vi "Parsing_TheGooodOne.vi"(6 "array":dbl[](array[numeric])=[0.0], 7 "Iterations":i32=6079, 8 "Search_Params":string[](array[string])=["B", "X", "Y", "W1", "H1", "W2", "H2"], 9 "Input":string="B:0,X:-3,Y:-3,W1:-3,H1:-3,W2:-3,H2:-3") -> (2 "Corrected distance":dbl=-10000.0, 3 "Value-Reference":dbl=-292.57472985881094)   [LabVIEW 2016]
uses:
  <vilib>/Analysis/3filter.llb/IIR Filter (DBL).vi
  <vilib>/Analysis/NI_AALBase.lvlib
panel:
  in  "Bad Value Count":i32=4
  out "Waveform Chart":cluster{dbl, dbl}(graph)={-10000.0, -292.57472985881094}
  out "Positions 2":i32[](array[numeric])
  out "Distance":dbl=133.35829999999999
  out "Move left":bool
  out "Move right":bool
  out "Not target":bool=TRUE
  in  "Desired_Midpoint":i32=200
  in  "High_Band":i32=10
  in  "Low_Band":i32=10
  out "Error":i32
  in  "P-gain":dbl format="%#_13g"
  out "Effort_Error":dbl
  out "Good_Midp":bool
  out "X Value":i32
  out "Good Target 2":bool
  out "Positions":i32[](array[numeric])
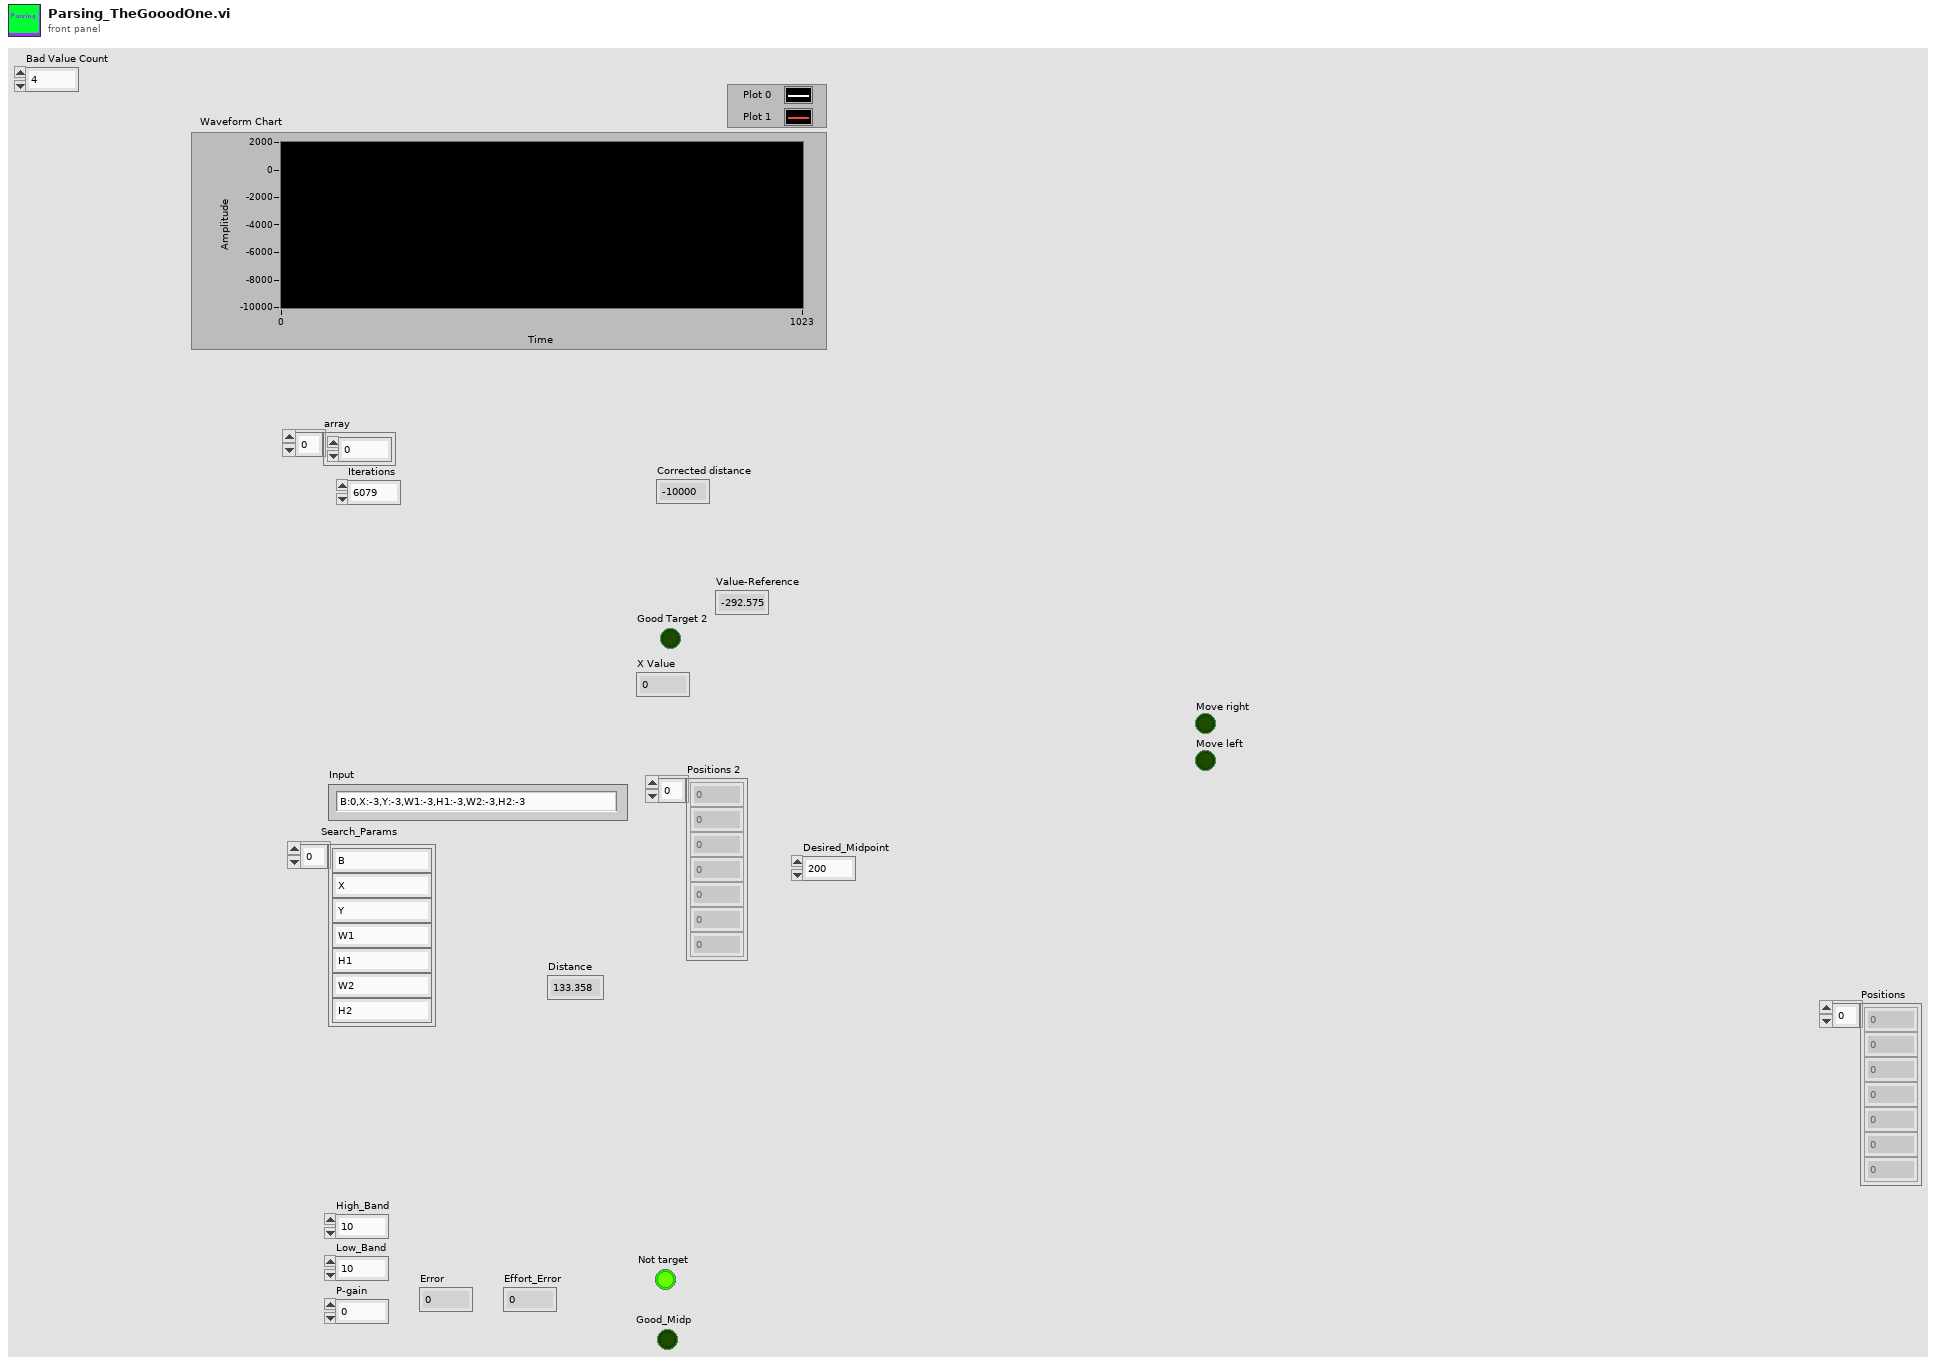
[diagram p1: front panel]
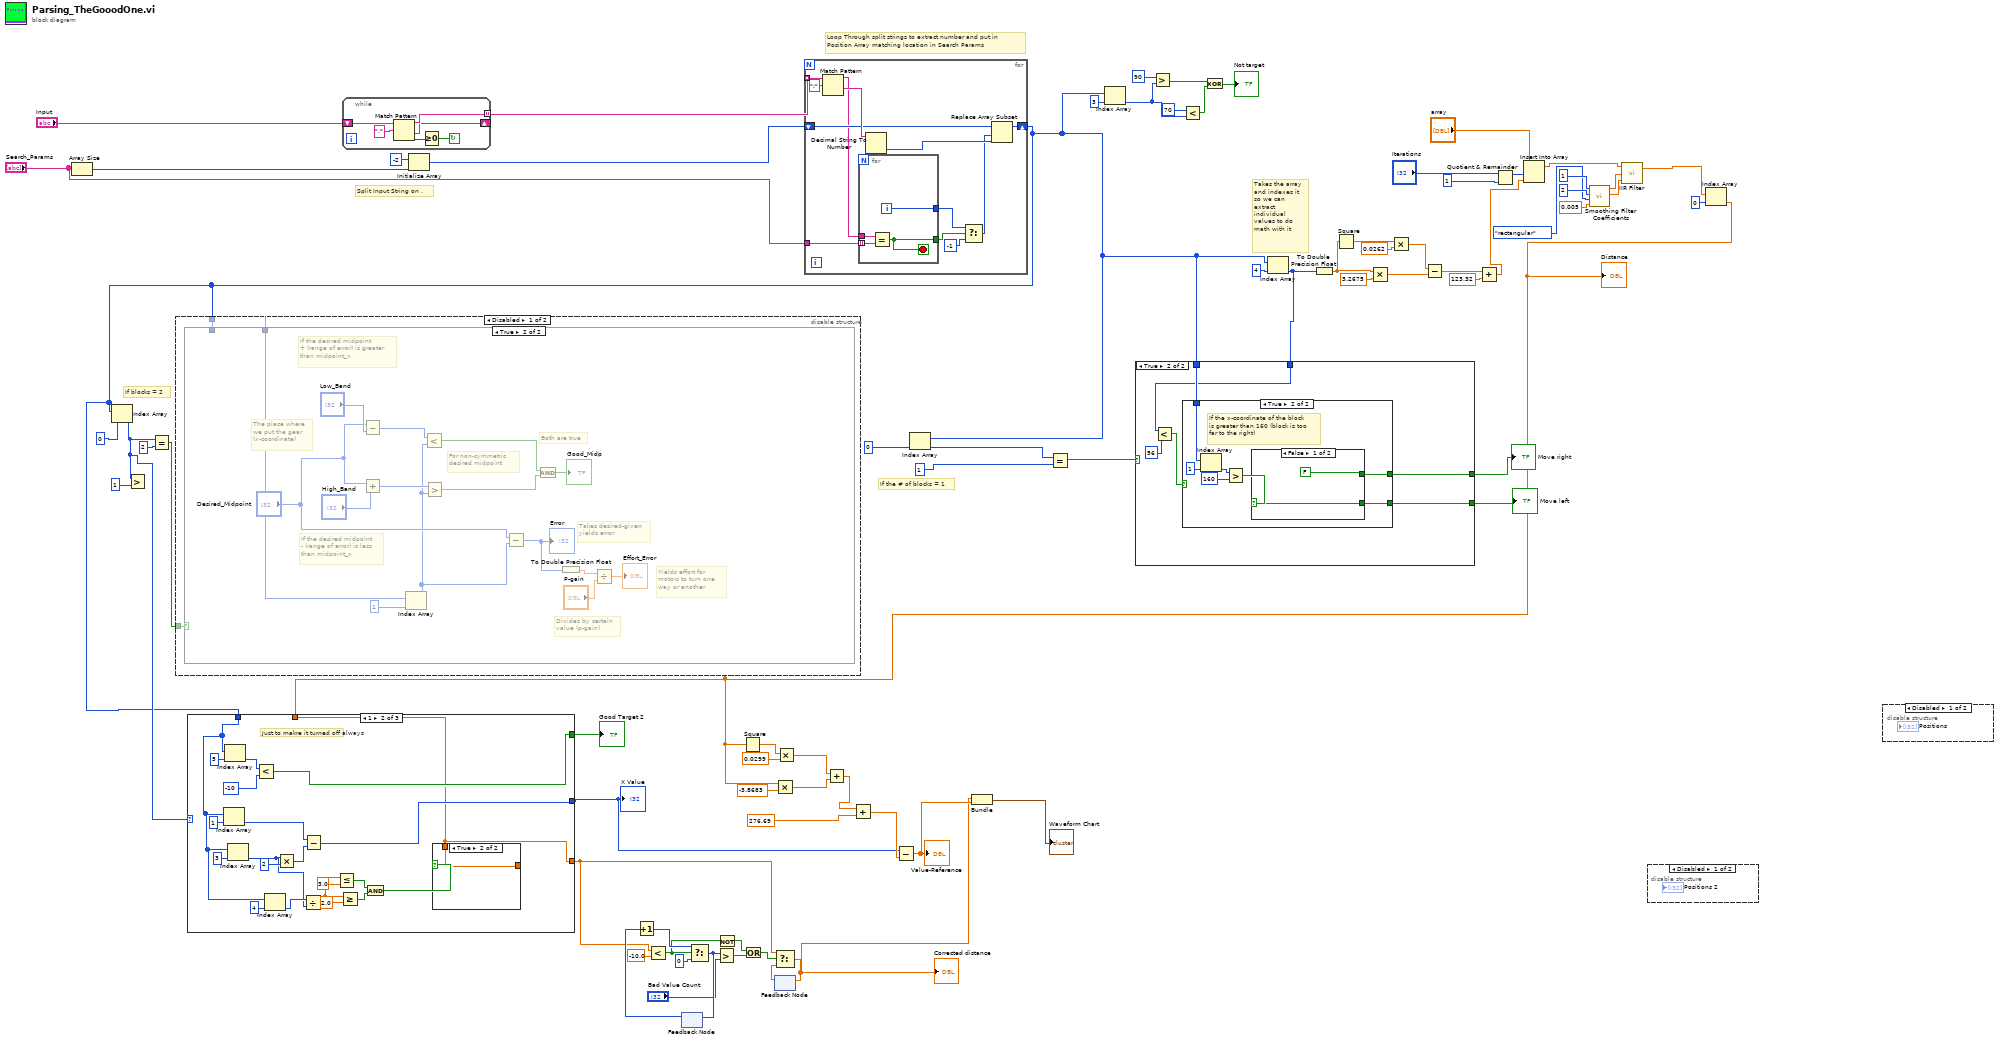
[diagram p0: block diagram]
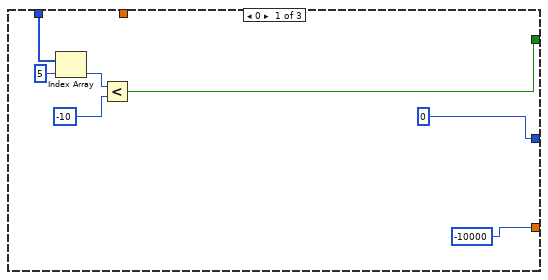
[diagram p2: hidden frame]
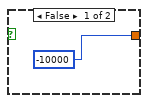
[diagram p3: hidden frame]
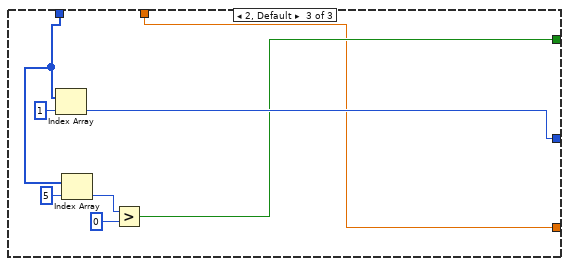
[diagram p4: hidden frame]
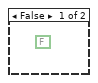
[diagram p5: hidden frame]
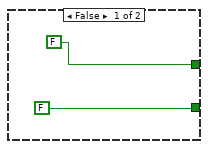
[diagram p7: hidden frame]
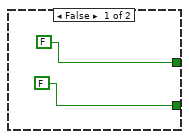
[diagram p8: hidden frame]
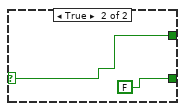
[diagram p9: hidden frame]
diagram:
  # "If blocks = 2"
  # "If the # of blocks = 1"
  # "Takes the array and indexes it so we can extract individual values to do math with it"
  # "Loop Through split strings to extract number and put in\nPosition Array matching location in Search Params"
  # "Split Input String on ,"
  n1 = Array Size(array="Search_Params") -> (size(s)=w36:i32)
  n2 = while {
    shift-right: [w78] -> _
    shift-left: "Input" -> [w81]
    tunnel: [w79] -> w32 mode=indexing
    stop <- w76 continue-if-true
    n3 = Match Pattern(string=w81, regular expression=",") -> (before substring=w79:string, after substring=w78:string, offset past match=w77:i32)  [unwired: 1 in, 1 out]
    n4 = Greater Or Equal To 0?(x=w77) -> (x >= 0?=w76:bool)
  }
  n5 = Initialize Array(-2 ("element"), w36) -> (w34:i32[])
  n6 = feedback #1() -> (w11:i32)  [unwired: 1 in]
  n7 = Increment(x=w11) -> (x+1=w12:i32)
  n8 = feedback #2() -> (w4:dbl)  [unwired: 1 in]
  n9 = for {
    tunnel: w32 -> [w93] mode=indexing
    shift-right: [w89] -> w64
    shift-left: w34 -> [w90]
    tunnel: "Search_Params" -> [w86]
    n10 = Match Pattern(string=w93, regular expression=":") -> (before substring=w87:string, after substring=w91:string)  [unwired: 1 in, 2 out]
    n11 = for {
      tunnel: w87 -> [w97]
      tunnel: w86 -> [w96] mode=indexing
      tunnel: [w94] -> w85
      tunnel: [w95] -> w84
      i -> [w95]
      stop <- w94 stop-if-true
      n12 = Equal?(x=w97, y=w96) -> (x = y?=w94:bool)
    }
    n13 = Decimal String To Number(string=w91) -> (number=w88:i32)  [unwired: 2 in, 1 out]
    n14 = Select(t=w84, s=w85, f=-1) -> (s? t:f=w82:i32)
    n15 = Replace Array Subset(array=w90, new element=w88, index=w82) -> (w89:i32[])
  }
  n16 = Index Array(array=w64, index=0) -> (element=w65:i32)
  n17 = Greater?(x=w65, y=1) -> ()  [unwired: 1 out]
  n18 = Equal?(x=w65, y=2) -> (x = y?=w55:bool)
  n19 = disable-structure shown="Disabled" {
    disable-tunnel: w55 -> [w99 _]
    disable-tunnel: w64 -> [w98 _]
    frame Disabled {
      n20 = case shown="True" w99 {
        tunnel: w98 -> [_ _]
        tunnel: w98 -> [_ w100]
        frame False {
          (unwired) FALSE
        }
        frame True {
          # "Yields effort for\nmotors to turn one\nway or another"
          # "Divides by certain\nvalue (p-gain)"
          # "Takes desired-given\nyields error"
          # "The place where\nwe put the gear \n(x-coordinate)"
          # "Both are true"
          # "For non-symmetric\ndesired midpoint"
          # "If the desired midpoint\n- (range of error) is less\nthan midpoint_x"
          # "If the desired midpoint\n+ (range of error) is greater\nthan midpoint_x"
          n21 = Subtract(x="Desired_Midpoint", y="Low_Band") -> (x-y=w110:i32)
          n22 = Add(x="Desired_Midpoint", y="High_Band") -> (x+y=w111:i32)
          n23 = Index Array(array=w100, index=1) -> (element=w106:i32)
          n24 = Less?(x=w110, y=w106) -> (x < y?=w109:bool)
          n25 = Greater?(x=w111, y=w106) -> (0:w108:bool)
          n26 = Subtract(x="Desired_Midpoint", y=w106) -> (x-y=w105:i32)
          "Error" <- w105
          n27 = And(x=w109, y=w108) -> (x .and. y?=→"Good_Midp":bool)
          n28 = To Double Precision Float(number=w105) -> (double precision float=w104:dbl)
          n29 = Divide(x=w104, y="P-gain") -> (x/y=→"Effort_Error":dbl)
        }
      }
    }
    frame Enabled {
    }
  }
  n30 = Index Array(array=w64, index=0) -> (element=w47:i32)
  n31 = Equal?(x=w47, y=1) -> (x = y?=w49:bool)
  n32 = Index Array(array=w64, index=3) -> (element=w58:i32)
  n33 = Greater?(x=90, y=w58) -> (0:w60:bool)
  n34 = Less?(x=70, y=w58) -> (x < y?=w61:bool)
  n35 = Exclusive Or(1:w61, 2:w60) -> (0:→"Not target":bool)
  n36 = Index Array(array=w64, index=4) -> (element=w50:i32)
  n37 = case shown="True" w49 {
    tunnel: w64 -> [_ w122]
    tunnel: w50 -> [_ w120]
    tunnel: [FALSE w118] -> w51
    tunnel: [FALSE w117] -> w52
    frame False {
    }
    frame True {
      n38 = Less?(x=w120, y=56) -> (x < y?=w119:bool)
      n39 = case shown="True" w119 {
        tunnel: w122 -> [_ w131]
        tunnel: [FALSE w126] -> w118
        tunnel: [FALSE w125] -> w117
        frame False {
        }
        frame True {
          # "If the x-coordinate of the block\nis greater than 160 (block is too\nfar to the right)"
          n40 = Index Array(array=w131, index=1) -> (element=w129:i32)
          n41 = Greater?(x=w129, y=160) -> (0:w127:bool)
          n42 = case shown="False" w127 {
            selector: w127 -> [w133 w135]
            tunnel: [w133 FALSE] -> w126
            tunnel: [FALSE w135] -> w125
            frame False {
            }
            frame True {
            }
          }
        }
      }
    }
  }
  "Move left" <- w51
  "Move right" <- w52
  n43 = To Double Precision Float(number=w50) -> (double precision float=w40:dbl)
  n44 = Square(x=w40) -> (x^2=w38:dbl)
  n45 = Multiply(x=w40, y=3.2675) -> (x*y=w42:dbl)
  n46 = Multiply(x=w38, y=0.0262) -> (x*y=w39:dbl)
  n47 = Subtract(x=w39, y=w42) -> (x-y=w43:dbl)
  n48 = Add(x=w43, y=123.32) -> (x+y=w18:dbl)
  n49 = Quotient & Remainder(x="Iterations", y=1) -> (x-y*floor(x/y)=w25:i32)  [unwired: 1 out]
  n50 = Insert Into Array(array="array", index=w25, new element=w18) -> (w19:dbl[])
  n51 = call <vilib>:"Smoothing Filter Coefficients.vi"("time constant"=0.005, "shape"=enum16{"rectangular", "triangular"}."rectangular", "half-width"=2, "type"=1) -> ("forward coefficients"=w26:dbl[], "reverse coefficients"=w27:dbl[])  [unwired: 5 in, 1 out]
  n52 = call-poly <vilib>:"IIR Filter.vi"("Forward Coefficients"=w26, "Reverse Coefficients"=w27, "X"=w19) -> ("Filtered X"=w24:dbl[])  [unwired: 1 in, 1 out]
  n53 = disable-structure shown="Disabled" {
    frame Disabled {
    }
    frame Enabled {
    }
  }
  n54 = Index Array(array=w24, index=0) -> (element=w17:dbl)
  "Distance" <- w17
  n55 = case shown="1" w65 {
    tunnel: w64 -> [w139 w153 w172]
    tunnel: w17 -> [_ w143 w166]
    tunnel: [0 w155 w168] -> w74
    tunnel: [w137 w154 w167] -> w66
    tunnel: [-10000 w143 w166] -> w5
    frame 0 {
      n56 = Index Array(array=w139, index=5) -> (element=w141:i32)
      n57 = Less?(x=w141, y=-10) -> (x < y?=w137:bool)
    }
    frame 1 {
      # "Just to makre it turned off always"
      n58 = Index Array(array=w153, index=1) -> (element=w156:i32)
      n59 = Index Array(array=w153, index=5) -> (element=w161:i32)
      n60 = Index Array(array=w153, index=3) -> (element=w150:i32)
      n61 = Less?(x=w161, y=-10) -> (x < y?=w154:bool)
      n62 = Index Array(array=w153, index=4) -> (element=w151:i32)
      n63 = Multiply(x=w150, y=2) -> (x*y=w157:i32)
      n64 = Divide(x=w151, y=w150) -> (x/y=w149:dbl)
      n65 = Subtract(x=w156, y=w157) -> (x-y=w155:i32)
      n66 = Less Or Equal?(x=w149, y=3.0) -> (x <= y?=w145:bool)
      n67 = Greater Or Equal?(x=w149, y=2.0) -> (x >= y?=w146:bool)
      n68 = And(x=w145, y=w146) -> (x .and. y?=w144:bool)
      n69 = case shown="True" w144 {
        tunnel: w143 -> [_ w165]
        tunnel: [-10000 ("y") w165] -> _
        frame False {
        }
        frame True {
        }
      }
    }
    frame 2, Default {
      n70 = Index Array(array=w172, index=1) -> (element=w168:i32)
      n71 = Index Array(array=w172, index=5) -> (element=w170:i32)
      n72 = Greater?(x=w170, y=0) -> (0:w167:bool)
    }
  }
  "X Value" <- w74
  "Good Target 2" <- w66
  n73 = Less?(x=w5, y=-10.0) -> (x < y?=w7:bool)
  n74 = Select(t=w12, s=w7, f=0) -> (s? t:f=w10:i32)
  n75 = feedback-in #1(w10) -> ()
  n76 = Greater?(x=w10, y="Bad Value Count") -> (0:w8:bool)
  n77 = Not(x=w7) -> (.not. x?=w1:bool)
  n78 = Square(x=w17) -> (x^2=w67:dbl)
  n79 = Or(x=w1, y=w8) -> (x .or. y?=w6:bool)
  n80 = Multiply(x=w17, y=-3.8683) -> (x*y=w71:dbl)
  n81 = Select(t=w5, s=w6, f=w4) -> (s? t:f=w3:dbl)
  "Corrected distance" <- w3
  n82 = feedback-in #2(w3) -> ()
  n83 = Multiply(x=w67, y=0.0299) -> (x*y=w70:dbl)
  n84 = Add(x=w70, y=w71) -> (x+y=w73:dbl)
  n85 = Add(x=w73, y=276.69) -> (x+y=w75:dbl)
  n86 = Subtract(x=w74, y=w75) -> (x-y=w15:dbl)
  "Value-Reference" <- w15
  n87 = Bundle(w3, w15) -> (→"Waveform Chart":cluster{dbl, dbl})  [unwired: 1 in]
  n88 = disable-structure shown="Disabled" {
    frame Disabled {
    }
    frame Enabled {
    }
  }
